vi "ParseArguments.vi"(11 "Arguments":string[](array[string])) -> (1 "Output Path":path, 2 "New VI Path":path, 3 "Old VI Path":path, 5 "Boolean":bool)   [LabVIEW 2017]
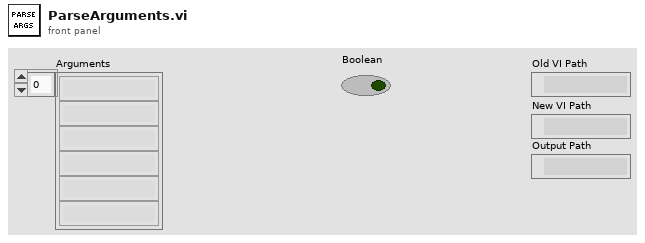
[diagram p1: front panel]
types:
  T1 = cluster{"Old VI Path":path, "New VI Path":path, "Output Path":path}
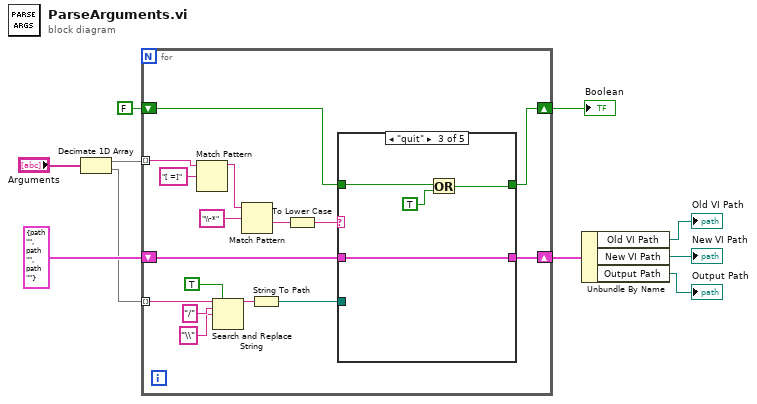
[diagram p0: block diagram]
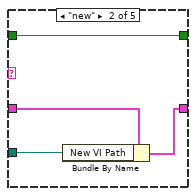
[diagram p3: hidden frame]
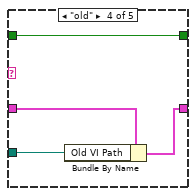
[diagram p4: hidden frame]
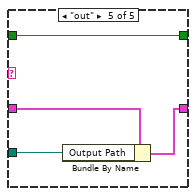
[diagram p5: hidden frame]
diagram:
  n1 = Decimate 1D Array("Arguments") -> (w4:string[], w3:string[])
  n2 = for {
    tunnel: w4 -> [w26] mode=indexing
    shift-right: [w14] -> w9
    shift-left: T1 {"Old VI Path"=path "", "New VI Path"=path "", "Output Path"=path ""} ("Expected Values") -> [w15]
    tunnel: w3 -> [w13] mode=indexing
    shift-right: [w12] -> w2
    shift-left: FALSE -> [w11]
    n3 = Match Pattern(string=w26, regular expression="[ =]") -> (before substring=w24:string)  [unwired: 1 in, 3 out]
    n4 = Search and Replace String(replace all?=TRUE ("replace all? (F)"), input string=w13, search string="/", replace string="\\" ("search string")) -> (result string=w17:string)  [unwired: 4 in, 3 out]
    n5 = Match Pattern(string=w24, regular expression="\\-*") -> (after substring=w22:string)  [unwired: 1 in, 3 out]
    n6 = String To Path(string=w17) -> (path=w16:path)
    n7 = To Lower Case(string=w22) -> (all lower case string=w21:string)
    n8 = case shown="\"quit\"" w21 {
      tunnel: w16 -> [_ w31 _ w39 w43]
      tunnel: w15 -> [w28 w32 w33 w40 w44]
      tunnel: [w28 w30 w33 w38 w42] -> w14
      tunnel: [w27 w29 w35 w37 w41] -> w12
      tunnel: w11 -> [w27 w29 w36 w37 w41]
      frame Default {
        # "Ignore other arguments"
      }
      frame "new" {
        n9 = Bundle By Name(cluster=w32, "New VI Path"=w31) -> (w30:T1)
      }
      frame "quit" {
        n10 = Or(x=w36, y=TRUE) -> (x .or. y?=w35:bool)
      }
      frame "old" {
        n11 = Bundle By Name(cluster=w40, "Old VI Path"=w39) -> (w38:T1)
      }
      frame "out" {
        n12 = Bundle By Name(cluster=w44, "Output Path"=w43) -> (w42:T1)
      }
    }
  }
  "Boolean" <- w2
  n13 = Unbundle By Name(w9) -> ("Old VI Path"=→"Old VI Path":path, "New VI Path"=→"New VI Path":path, "Output Path"=→"Output Path":path)
